vi "Do.vi"(8 "error in (no error)":errorcluster, 10 "Actor in":refnum<class "Actor.lvclass">, 11 "Update Point Data Msg":refnum<class "Update Point Data Msg.lvclass">) -> (0 "error out":errorcluster, 2 "Actor out":refnum<class "Actor.lvclass">)   [LabVIEW 2024, in "ITask Actor.lvlib" / "Update Point Data Msg.lvclass"]
doc: "This VI delivers the message to the actor by calling the appropriate method(s) on the actor."
uses:
  Update Point Data Msg.lvclass
  <vilib>/ActorFramework/Actor/Actor.lvclass
  Update Point Data Msg.lvclass/Update Point Data Msg.ctl
  ITask Actor/ITask Actor.lvclass
  9ef47adc-f318-494c-9b8b-6df3216d6863.vi
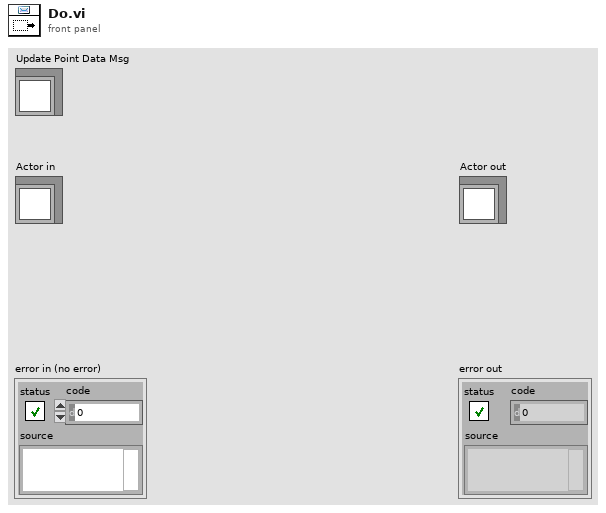
[diagram p1: front panel]
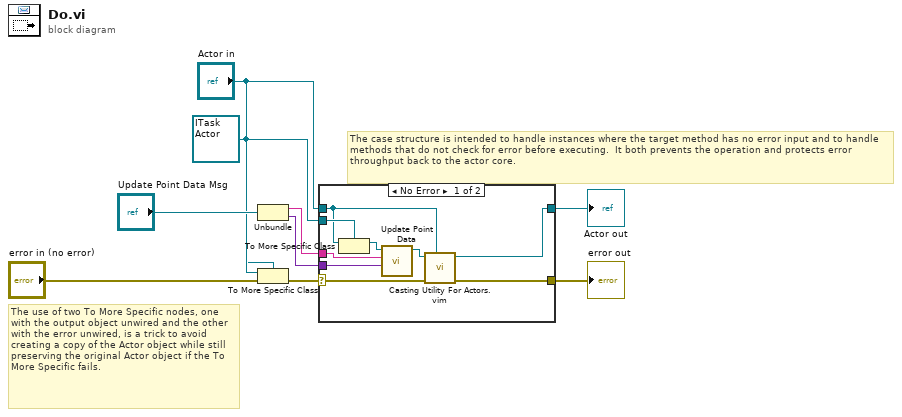
[diagram p0: block diagram]
diagram:
  w3 = refnum<class "ITask Actor.lvclass"> refnum ("Actor in")
  # "The use of two To More Specific nodes, one with the output object unwired and the other with the error unwired, is a trick to avoid creating a copy of the Actor object while still preserving the original Actor object if the To More Specific fails."
  # "The case structure is intended to handle instances where the target method has no error input and to handle methods that do not check for error before executing.  It both prevents the operation and protects error throughput back to the actor core."
  n1 = Unbundle("Update Point Data Msg") -> (w2:string, w1:variant)
  n2 = To More Specific Class(target class=w3, reference="Actor in", error in="error in (no error)") -> (error out=w7:errorcluster)  [unwired: 1 out]
  n3 = case shown="No Error" w7 {
    selector: w7 -> [w18 w20]
    tunnel: [w12 w20] -> w6
    tunnel: [w13 w19] -> w5
    tunnel: "Actor in" -> [w15 w19]
    tunnel: w3 -> [w16 _]
    tunnel: w2 -> [w11 _]
    tunnel: w1 -> [w10 _]
    frame No Error {
      n4 = To More Specific Class(target class=w16, reference=w15) -> (specific class reference=w17:refnum<class "ITask Actor.lvclass">)  [unwired: 1 in, 1 out]
      n5 = call-dynamic "Update Point Data.vi"("Data"=w10, "Point Ident"=w11, "ITask Actor in"=w17) -> ("ITask Actor out"=w14:refnum<class "ITask Actor.lvclass">)  [unwired: 8 in]
      n6 = call "Casting Utility For Actors.vim"("type"=w15, "error in (no error)"=w18, "Actor in"=w14) -> ("error out"=w12:errorcluster, "Actor out"=w13:refnum<class "Actor.lvclass">)  [unwired: 7 in]
    }
    frame Error {
      # "If type check fails, pass the original object out again."
    }
  }
  "error out" <- w6
  "Actor out" <- w5
